vi "count rate shift.vi"(7 "read or write":string(combo)="read", 10 "count rate in":dbl) -> (2 "count rate out":dbl)   [LabVIEW 2016]
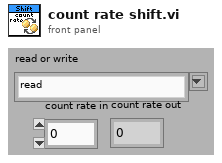
[diagram p1: front panel]
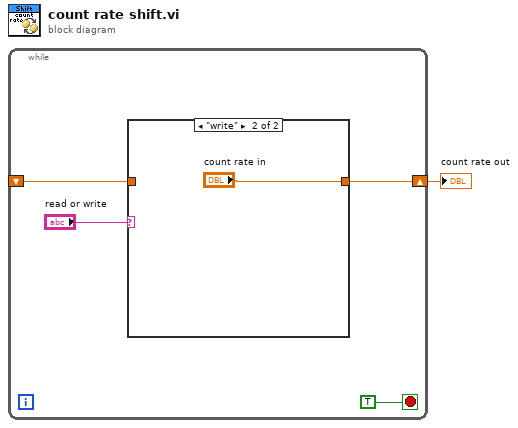
[diagram p0: block diagram]
diagram:
  n1 = while {
    shift-right: [w4] -> w1
    shift-left: _ -> [w3]
    stop <- TRUE stop-if-true
    n2 = case shown="\"write\"" "read or write" {
      tunnel: [w6 "count rate in"] -> w4
      tunnel: w3 -> [w6 _]
      frame "read", Default {
      }
      frame "write" {
      }
    }
  }
  "count rate out" <- w1
